vi "VisualizeStatus.vi"(10 "ModuleList":string[](array[string])=["Sync", "FGen", "Digitizer", "Sensor", "Analysis", "Scope", "AcPwr"]) -> ()   [LabVIEW 2018, in "Visualization.lvlib" / "VisualizeStatus.lvclass"]
uses:
  VisualizeStatus.lvclass
  VisualizeBase/VisualizeBase_class/SubVIs/VisualizationOptions.ctl
  <vilib>/Utility/miscctls.llb/LVRectTypeDef.ctl
  LV_Config_class/Config.lvclass/Config.ctl
  LV_Config_class/Typedefs/eLogLvl.ctl
  <vilib>/Utility/error.llb/DialogType.ctl
  VisualizeBase/VisualizeBase_class/Requests/VisUserEventType.ctl
  <vilib>/event_ctls.llb/usereventprio.ctl
  LV_Config_class/Accessors/Read ConfigFilePath.vi
  <extravilib>/ChannelInstances/Tag-bool/Write With Abort.vi
  <extravilib>/ChannelInstances/Tag-bool/Read With Abort.vi
  <vilib>/Utility/error.llb/Error Cluster From Error Code.vi
  <extravilib>/ChannelInstances/Tag-bool/Instantiate.vi
  <extravilib>/ChannelInstances/Tag-bool/EndpointRead.vi
  <userlib>/_OpenG.lib/string/string.llb/Convert EOLs (String)__ogtk.vi
  <extravilib>/ChannelInstances/Tag-bool/Endpoint.vi
  <vilib>/ErrorRing/Error Ring.xnode
  <userlib>/NIST/NISTErrorLib/NISTErrorLib.lvlib
  VisualizeBase/VisualizeBase_class/VisualizeBase.lvclass
  Sync/SyncModule/SyncModule.lvlib
  Digitizer/DigitizerModule/DigitizerModule.lvlib
  BusClass/Bus.lvclass
  Sensor/SensorModule/SensorModule.lvlib
  Analysis/AnalysisModule/AnalysisModule.lvlib
  Scope/ScopeModule/ScopeModule.lvlib
  AcPwr/AcPwrShared/AcPwrShared.lvlib
  <extravilib>/ChannelInstances/Tag-bool.lvlib
  TestClass/Test.lvclass
  FGen/FgenShared/FgenShared.lvlib
  LV_Config_class/Config.lvclass
panel:
  in  "Text.Scroll Position":i32=-1
  out "VisualizationProperties":T1={"PauseAtStartup"=TRUE, "LogData"=FALSE, "LaunchInSubPanel"=TRUE, "FPMonitor"=0, "FPWindowBounds"={"Left"=0, "Top"=0, "Right"=0, "Bottom"=0}, "MonitorBounds"={"Left"=0, "Top"=0, "Right"=0, "Bottom"=0}, "MeasIndices"=[]}
  out "Status Message":string
  in  "INIFilePath":path
  in  "Log Data":bool
  out "ErrorArray":errorcluster[](array[cluster])
  in  "btnRestart":bool
  in  "btnPause":bool
  in  "btnReset":bool
  in  "btnClear":bool
  in  "btnStop&Exit":bool
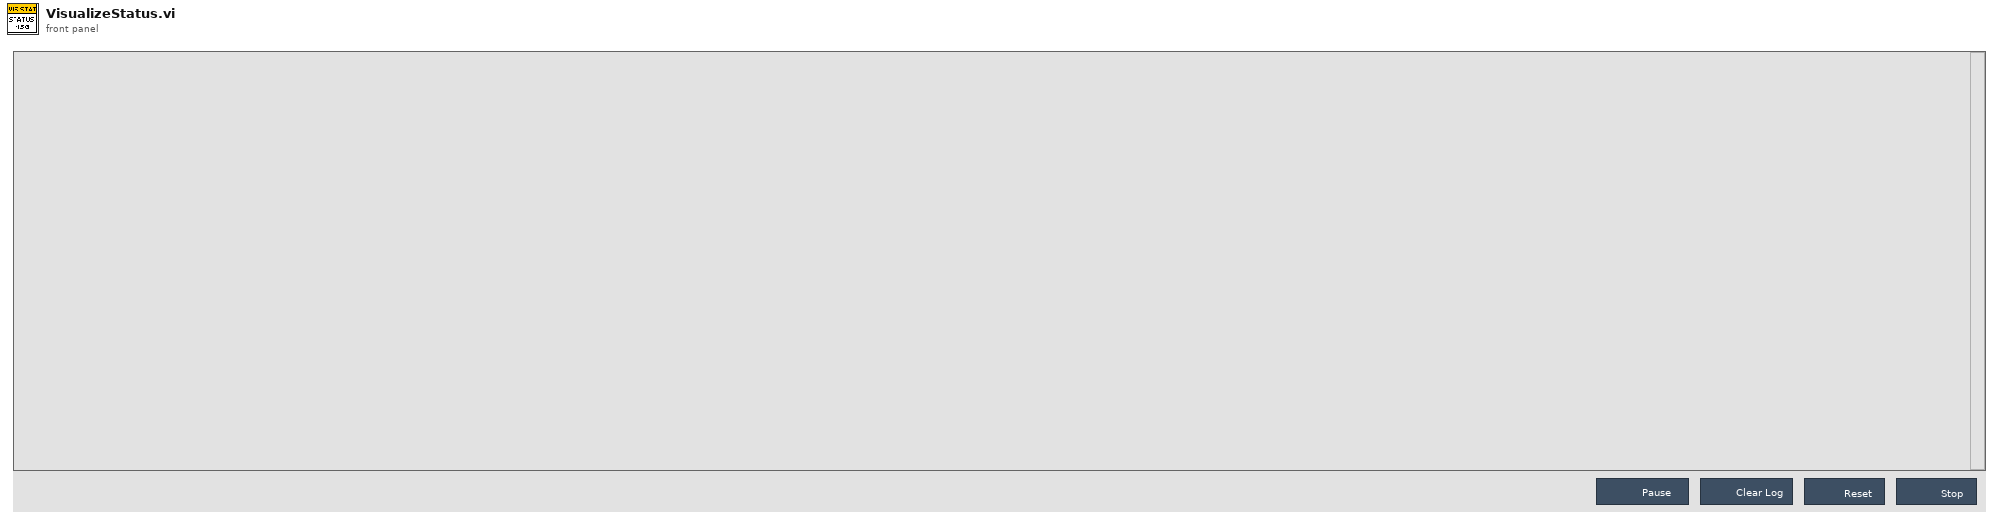
[diagram p1: front panel]
types:
  T1 = typedef "Visualization.lvlib/VisualizeBase.lvclass/VisualizationOptions.ctl" = cluster{"PauseAtStartup":bool, "LogData":bool, "LaunchInSubPanel":bool, "FPMonitor":u16, "FPWindowBounds":T2, "MonitorBounds":cluster{"Left":i16, "Top":i16, "Right":i16, "Bottom":i16}, "MeasIndices":i32[]}
  T2 = typedef "LVRectTypeDef.ctl" = cluster{"Left":i16, "Top":i16, "Right":i16, "Bottom":i16}
  T3 = typedef "SyncModule.lvlib/SyncBroadcastEvents.ctl" = cluster{"DidInit":refnum<user-event>, "StatusUpdate":refnum<user-event>, "ErrorReport":refnum<user-event>, "DidStop":refnum<user-event>, "PathToINI":refnum<user-event>, "TriggerTime":refnum<user-event>, "LockStatus":refnum<user-event>, "Info":refnum<user-event>, "ClockProperties":refnum<user-event>, "SyncData":refnum<user-event>, "TimingSession":refnum<user-event>}
  T4 = typedef "AcPwrShared.lvlib/AcPwrBroadcastEvents.ctl" = cluster{"DidInit":refnum<user-event>, "StatusUpdate":refnum<user-event>, "ErrorReport":refnum<user-event>, "DidStop":refnum<user-event>, "PathToINI":refnum<user-event>, "Measurements":refnum<user-event>, "LoadConfigFile":refnum<user-event>, "GetSettings":refnum<user-event>, "SetSettings":refnum<user-event>, "GetType&ID":refnum<user-event>, "GotSettings":refnum<user-event>, "GotSettingsLV":refnum<user-event>, "ParameterSet":refnum<user-event>}
  T5 = typedef "FgenShared.lvlib/clBroadcastEvents.ctl" = cluster{"DidInit":refnum<user-event>, "StatusUpdate":refnum<user-event>, "ErrorReport":refnum<user-event>, "DidStop":refnum<user-event>, "PathToINI":refnum<user-event>, "Channels":refnum<user-event>, "Function":refnum<user-event>, "Waveforms":refnum<user-event>, "Triggers":refnum<user-event>, "FunctionParams":refnum<user-event>, "FunctionArbs":refnum<user-event>, "FunctionSampleRate":refnum<user-event>}
  T6 = typedef "ScopeShared.lvlib/clBroadcastEvents.ctl" = cluster{"DidInit":refnum<user-event>, "StatusUpdate":refnum<user-event>, "ErrorReport":refnum<user-event>, "DidStop":refnum<user-event>, "PathToINI":refnum<user-event>, "Handle":refnum<user-event>, "Model":refnum<user-event>, "Channels":refnum<user-event>, "Acquisition":refnum<user-event>, "Trigger":refnum<user-event>, "ExtAcquisition":refnum<user-event>, "Waveform":refnum<user-event>}
  T7 = typedef "DigitizerShared.lvlib/clBroadcastEvents.ctl" = cluster{"DidInit":refnum<user-event>, "StatusUpdate":refnum<user-event>, "ErrorReport":refnum<user-event>, "DidStop":refnum<user-event>, "PathToINI":refnum<user-event>, "Channels":refnum<user-event>, "Acq":refnum<user-event>, "Trigger":refnum<user-event>, "Waveforms":refnum<user-event>}
  T8 = typedef "SensorShared.lvlib/clBroadcastEvents.ctl" = cluster{"DidInit":refnum<user-event>, "StatusUpdate":refnum<user-event>, "ErrorReport":refnum<user-event>, "DidStop":refnum<user-event>, "PathToINI":refnum<user-event>, "SensorReport":refnum<user-event>, "SensorConfig":refnum<user-event>}
  T9 = typedef "AnalysisModule.lvlib/clBroadcastEvents.ctl" = cluster{"DidInit":refnum<user-event>, "StatusUpdate":refnum<user-event>, "ErrorReport":refnum<user-event>, "DidStop":refnum<user-event>, "PathToINI":refnum<user-event>, "Config":refnum<user-event>, "ResultReport":refnum<user-event>, "FunctionClass":refnum<user-event>, "State":refnum<user-event>, "FunctionParams":refnum<user-event>, "Duration":refnum<user-event>}
  T10 = cluster{"DigitizerEvents":T7, "FGenEvents":T5, "SyncBroadcastEvents":T3, "AnalysisBroadcastEvents":T9, "SensorBdcstEvents":T8, "ScopeEvents":T6, "clAcPwrEvents":T4}
  T11 = typedef "Visualization.lvlib/VisualizeBase.lvclass/VisRequestEvents.ctl" = cluster{"StopRequest":refnum<user-event>, "ResetRequest":refnum<user-event>, "FP Pop In or Out":refnum<user-event>}
  T12 = cluster{"StatusUpdate":refnum<user-event>, "ErrorReport":refnum<user-event>, "StatusUpdate":refnum<user-event>, "ErrorReport":refnum<user-event>, "StatusUpdate":refnum<user-event>, "ErrorReport":refnum<user-event>, "StatusUpdate":refnum<user-event>, "ErrorReport":refnum<user-event>, "StatusUpdate":refnum<user-event>, "ErrorReport":refnum<user-event>, "StatusUpdate":refnum<user-event>, "ErrorReport":refnum<user-event>, "FunctionClass":refnum<user-event>, "StatusUpdate":refnum<user-event>, "ErrorReport":refnum<user-event>}
  T13 = typedef "Visualization.lvlib/VisualizeBase.lvclass/VisFrmWrkBroadcastEvents.ctl" = cluster{"StatusUpdate":refnum<user-event>, "DidStop":refnum<user-event>, "NewModuleLoaded":refnum<user-event>, "StopVisualization":refnum<user-event>}
  T14 = typedef "Visualization.lvlib/VisualizeBase.lvclass/VisUserEventType.ctl" = cluster{"BusIndex":i8, "Data":variant}
  T15 = typedef "usereventprio.ctl" = enum32{"high priority", "normal priority"}
  T16 = typedef "Tag-bool.lvlib/))Channel.ctl" = refnum<queue>
  T17 = typedef "Config_class.lvlib/Config.lvclass/eLogLvl.ctl" = enum16{"Normal", "Verbose", "None"}
  T18 = typedef "DialogType.ctl" = u16
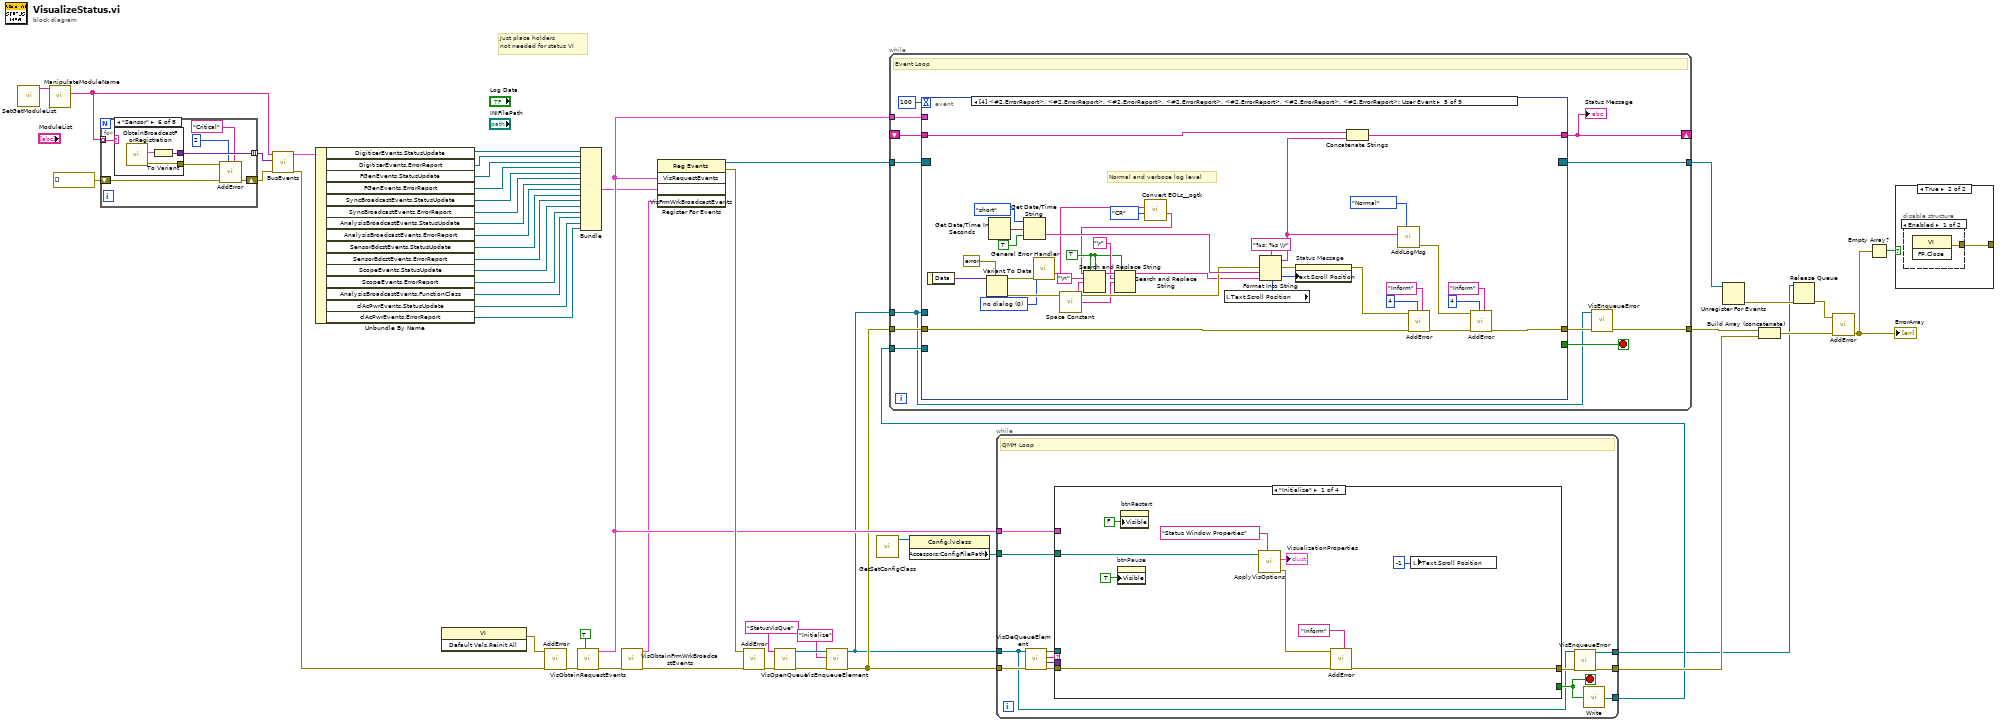
[diagram p0: block diagram]
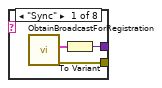
[diagram p2: hidden frame]
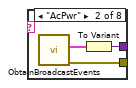
[diagram p3: hidden frame]
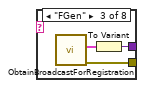
[diagram p4: hidden frame]
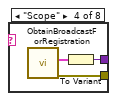
[diagram p5: hidden frame]
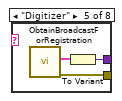
[diagram p6: hidden frame]
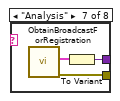
[diagram p7: hidden frame]
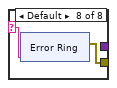
[diagram p8: hidden frame]
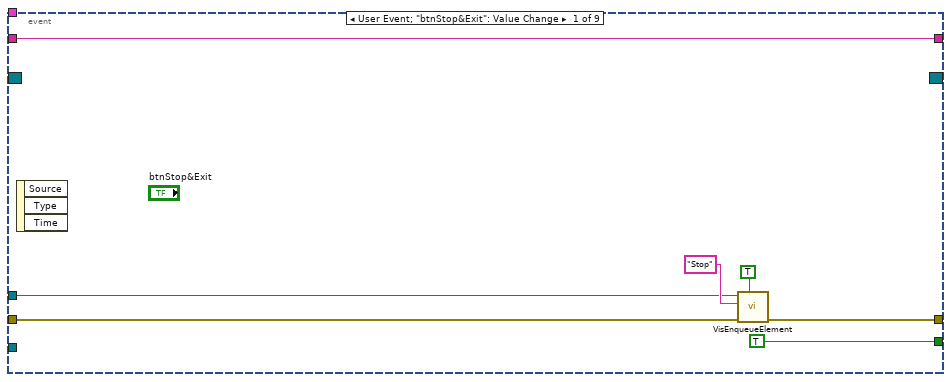
[diagram p9: hidden frame]
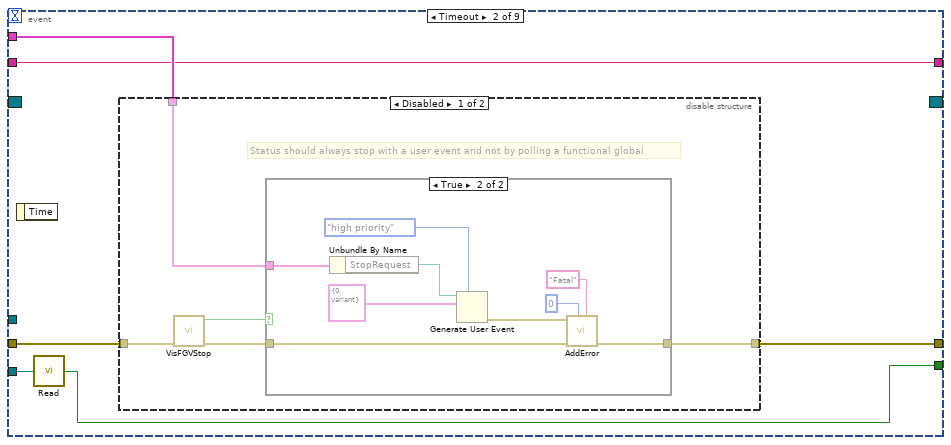
[diagram p10: hidden frame]
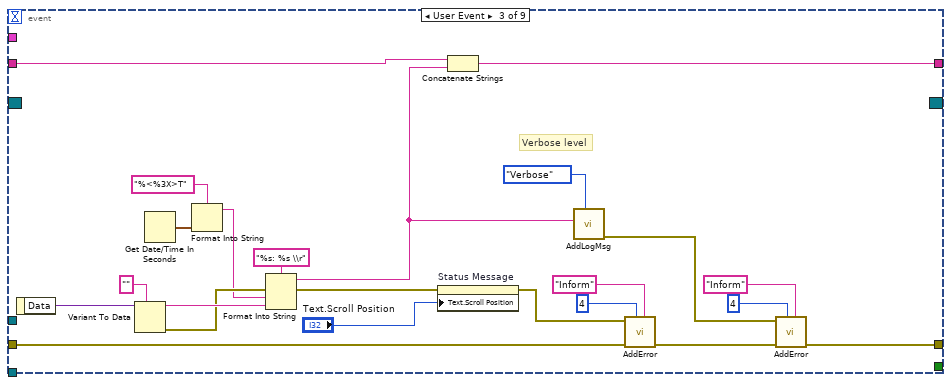
[diagram p13: hidden frame]
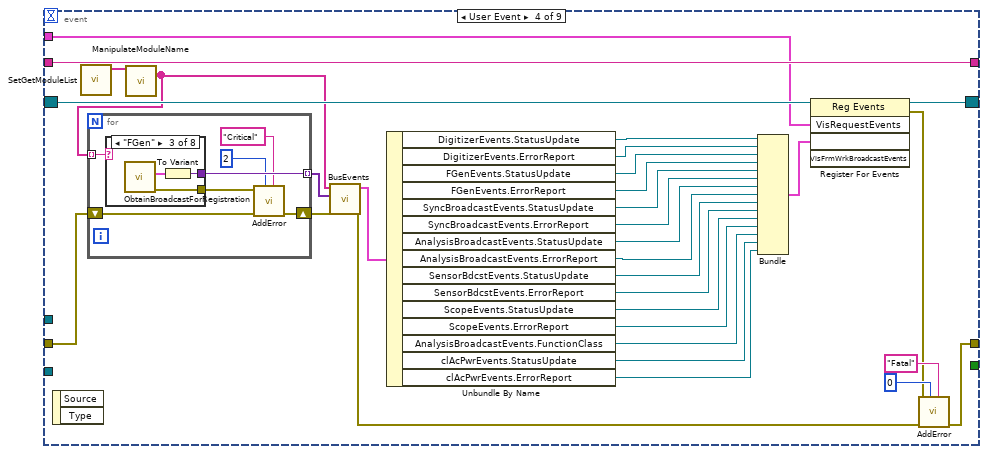
[diagram p14: hidden frame]
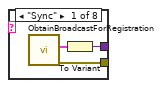
[diagram p15: hidden frame]
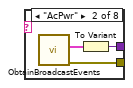
[diagram p16: hidden frame]
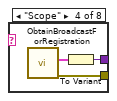
[diagram p17: hidden frame]
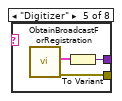
[diagram p18: hidden frame]
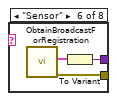
[diagram p19: hidden frame]
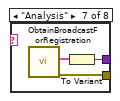
[diagram p20: hidden frame]
diagram:
  # "Just place holders\nnot needed for status VI"
  n1 = call "SetGetModuleList.vi"() -> ("ModuleList"=w35:string[])  [unwired: 11 in]
  n2 = call "ManipulateModuleName.vi"("ModuleListArrayIn"=w35) -> ("BeforeMatch:ModuleListArray"=w31:string[])  [unwired: 9 in, 5 out]
  n3 = for {
    shift-right: [w56] -> w33
    shift-left: errorcluster[] [] ("ErrorArray") -> [w55]
    tunnel: [w54] -> w32 mode=indexing
    tunnel: w31 -> [w51] mode=indexing
    n4 = case shown="\"Sensor\"" w51 {
      selector: w51 -> [_ _ _ _ _ _ _ w79]
      tunnel: [w59 w63 w65 w67 w71 w74 w77 _] -> w54
      tunnel: [w58 w62 w66 w69 w72 w75 w78 w80] -> w57
      frame "Sync" {
        n5 = call "ObtainBroadcastForRegistration.vi"() -> ("error out"=w58:errorcluster, "SyncBroadcastEvents"=w60:T3)  [unwired: 10 in]
        n6 = To Variant(anything=w60) -> (Variant=w59:variant)
      }
      frame "AcPwr" {
        n7 = call "ObtainBroadcastEvents.vi"() -> ("error out"=w62:errorcluster, "AcPwrEvents"=w61:T4)  [unwired: 10 in]
        n8 = To Variant(anything=w61) -> (Variant=w63:variant)
      }
      frame "FGen" {
        n9 = call "ObtainBroadcastForRegistration.vi"() -> ("error out"=w66:errorcluster, "FgenBroadcastEvents"=w64:T5)  [unwired: 10 in]
        n10 = To Variant(anything=w64) -> (Variant=w65:variant)
      }
      frame "Scope" {
        n11 = call "ObtainBroadcastForRegistration.vi"() -> ("error out"=w69:errorcluster, "ScopeBroadcastEvents"=w68:T6)  [unwired: 10 in]
        n12 = To Variant(anything=w68) -> (Variant=w67:variant)
      }
      frame "Digitizer" {
        n13 = call "ObtainBroadcastForRegistration.vi"() -> ("error out"=w72:errorcluster, "clDigitizerBdcstEvents"=w70:T7)  [unwired: 10 in]
        n14 = To Variant(anything=w70) -> (Variant=w71:variant)
      }
      frame "Sensor" {
        n15 = call "ObtainBroadcastForRegistration.vi"() -> ("error out"=w75:errorcluster, "SensorBdcstEvents"=w73:T8)  [unwired: 10 in]
        n16 = To Variant(anything=w73) -> (Variant=w74:variant)
      }
      frame "Analysis" {
        n17 = call "ObtainBroadcastForRegistration.vi"() -> ("error out"=w78:errorcluster, "AnalysisBroadcastEvents"=w76:T9)  [unwired: 10 in]
        n18 = To Variant(anything=w76) -> (Variant=w77:variant)
      }
      frame Default {
        n19 = xnode "Error Ring"("parameter 0"=w79) -> ("error out"=w80:errorcluster)
      }
    }
    n20 = call <userlib>:"AddError.vi"("Severity"="Critical", "Priority"=u8 2, "ErrorArray In"=w55, "error in (no error)"=w57) -> ("ErrorArray Out"=w56:errorcluster[])  [unwired: 6 in, 1 out]
  }
  n21 = call "BusEvents.vi"("Error in"=w33, "EventArray"=w32, "ModuleList"=w31) -> ("output cluster"=w30:T10)  [unwired: 7 in, 1 out]
  n22 = Unbundle By Name(w30) -> ("DigitizerEvents.StatusUpdate"=w29:refnum<user-event>, "DigitizerEvents.ErrorReport"=w28:refnum<user-event>, "FGenEvents.StatusUpdate"=w27:refnum<user-event>, "FGenEvents.ErrorReport"=w26:refnum<user-event>, "SyncBroadcastEvents.StatusUpdate"=w25:refnum<user-event>, "SyncBroadcastEvents.ErrorReport"=w24:refnum<user-event>, "AnalysisBroadcastEvents.StatusUpdate"=w23:refnum<user-event>, "AnalysisBroadcastEvents.ErrorReport"=w22:refnum<user-event>, "SensorBdcstEvents.StatusUpdate"=w21:refnum<user-event>, "SensorBdcstEvents.ErrorReport"=w20:refnum<user-event>, "ScopeEvents.StatusUpdate"=w19:refnum<user-event>, "ScopeEvents.ErrorReport"=w18:refnum<user-event>, "AnalysisBroadcastEvents.FunctionClass"=w17:refnum<user-event>, "clAcPwrEvents.StatusUpdate"=w16:refnum<user-event>, "clAcPwrEvents.ErrorReport"=w15:refnum<user-event>)
  n23 = invoke class="VI" method="Default Vals.Reinit All"() -> (error out=w50:errorcluster)  [unwired: 3 in, 2 out]
  n24 = call <userlib>:"AddError.vi"("ErrorArray In"=w33, "error in (no error)"=w50) -> ("ErrorArray Out"=w49:errorcluster[])  [unwired: 8 in, 1 out]
  n25 = call "VisObtainRequestEvents.vi"("Set (T)/Get (F)"=TRUE, "Error"=w49) -> ("Error"=w48:errorcluster[], "VisRequestEvents"=w36:T11)  [unwired: 8 in]
  n26 = Bundle("StatusUpdate"=w29, "ErrorReport"=w28, "StatusUpdate"=w27, "ErrorReport"=w26, "StatusUpdate"=w25, "ErrorReport"=w24, "StatusUpdate"=w23, "ErrorReport"=w22, "StatusUpdate"=w21, "ErrorReport"=w20, "StatusUpdate"=w19, "ErrorReport"=w18, "FunctionClass"=w17, "StatusUpdate"=w16, "ErrorReport"=w15) -> (w14:T12)  [unwired: 1 in]
  n27 = call "VisObtainFrmWrkBroadcastEvents.vi"("Error"=w48) -> ("Error"=w12:errorcluster[], "VisFrmWrkBroadcastEvents"=w11:T13)  [unwired: 9 in]
  n28 = register-events(w36, w14, w11) -> (reference out=w40:refnum<event-registration>, error out=w39:errorcluster)  [unwired: 2 in]
  n29 = call <userlib>:"AddError.vi"("ErrorArray In"=w12, "error in (no error)"=w39) -> ("ErrorArray Out"=w5:errorcluster[])  [unwired: 8 in, 1 out]
  n30 = call "VisOpenQueue.vi"("Error Array In"=w5, "QueueName"="StatusVisQue" ("QueName")) -> ("Error Array Out"=w7:errorcluster[], "queue out"=w8:refnum<queue>)  [unwired: 8 in]
  n31 = call "VisEnqueueElement.vi"("Error Array In"=w7, "Message"="Initialize", "queue in"=w8) -> ("Error Array Out"=w4:errorcluster[], "queue out"=w3:refnum<queue>)  [unwired: 7 in]
  n32 = call "GetSetConfigClass.vi"() -> ("Ref out"=w10:refnum<class "Config.lvclass">)  [unwired: 11 in]
  n33 = property class="Config.lvclass"(reference=w10) -> ("Accessors:ConfigFilePath"=w9:path)  [unwired: 1 in, 2 out]
  n34 = while {
    tunnel: w4 -> [w100]
    tunnel: [w94] -> w45
    tunnel: w36 -> [w93]
    tunnel: [w92] -> w37
    tunnel: w9 -> [w91]
    tunnel: w3 -> [w89]
    tunnel: [w88] -> w1
    stop <- w95 stop-if-true
    # "QMH Loop"
    n35 = call "VisDeQueueElement.vi"("Error Array In"=w100, "Queue In"=w89) -> ("Error Array Out"=w97:errorcluster[], "Data"=w98:variant, "Message"=w99:string, "Queue Out"=w90:refnum<queue>)  [unwired: 6 in]
    n36 = case shown="\"Initialize\"" w99 {
      selector: w99 -> [_ w117 _ _]
      tunnel: w98 -> [_ _ w132 _]
      tunnel: w97 -> [w110 w115 _ w164]
      tunnel: [w107 w114 w128 w162] -> w96
      tunnel: [_ _ w127 TRUE] -> w95
      tunnel: w93 -> [_ _ w126 _]
      tunnel: w91 -> [w109 _ _ w159]
      tunnel: w90 -> [_ _ w125 _]
      frame "Initialize" {
        n37 = property on="btnPause" class="Bool"("Visible"=TRUE) -> ()  [unwired: 2 in, 2 out]
        n38 = property on="btnRestart" class="Bool"("Visible"=FALSE) -> ()  [unwired: 2 in, 2 out]
        n39 = call "ApplyVisOptions.vi"("section (optional)"="Status Window Properties", "INIFilePath"=w109) -> ("error out"=w106:errorcluster, "VisualizationProperties"=→"VisualizationProperties":T1)  [unwired: 8 in]
        n40 = call <userlib>:"AddError.vi"("Severity"="Inform", "ErrorArray In"=w110, "error in (no error)"=w106) -> ("ErrorArray Out"=w107:errorcluster[])  [unwired: 7 in, 1 out]
        n41 = local write "Text.Scroll Position"(-1 ("Text.Scroll Position")) -> ()
      }
      frame Default {
        n42 = xnode "Error Ring"("parameter 0"=w117) -> ("error out"=w116:errorcluster)
        n43 = call <userlib>:"AddError.vi"("Severity"="Inform" ("String"), "Priority"=u8 5, "ErrorArray In"=w115, "error in (no error)"=w116) -> ("ErrorArray Out"=w114:errorcluster[], "error out"=w113:errorcluster)  [unwired: 6 in]
        n44 = call <vilib>:"Clear Errors.vi"("error in (no error)"=w113) -> ()  [unwired: 5 in, 2 out]
      }
      frame "Error" {
        n45 = Variant To Data(type=errorcluster[] [], Variant=w132) -> (data=w130:errorcluster[])  [unwired: 1 in, 1 out]
        n46 = call <userlib>:"ParseErrors.vi"("ErrorArray"=w130) -> ("ErrorArray"=w129:errorcluster[])  [unwired: 8 in, 2 out]
        n47 = for {
          tunnel: w129 -> [w143] mode=indexing
          tunnel: [w137] -> w128 mode=concatenating
          tunnel: [w135] -> w127
          tunnel: w126 -> [w134]
          tunnel: w125 -> [w133]
          stop <- w135 stop-if-true
          n48 = call <userlib>:"GeneralHandler.vi"("error in (no error)"=w143) -> ("Severity"=w136:string, "Stop"=w140:bool, "Abort"=w141:bool, "Continue"=w142:bool)  [unwired: 6 in, 1 out]
          n49 = Build Array(w142, w141, w140) -> (w139:bool[])
          n50 = Boolean Array To Number(Boolean array=w139) -> (number=w138:u32)
          n51 = case shown="2" w138 {
            tunnel: [_ _ w148 w156] -> w137
            tunnel: w136 -> [_ _ _ w152]
            tunnel: [_ _ _ w150] -> w135
            tunnel: w134 -> [_ _ _ w149]
            tunnel: w133 -> [_ _ w144 _]
            frame 0, Default {
              # "No Dialog"
            }
            frame 1 {
              # "Continue"
            }
            frame 2 {
              # "Abort, Flush Queue"
              n52 = Flush Queue(queue=w144) -> (error out=w147:errorcluster)  [unwired: 1 in, 2 out]
              n53 = call <userlib>:"AddError.vi"("Severity"="Critical" ("String"), "Priority"=u8 1, "error in (no error)"=w147) -> ("ErrorArray Out"=w148:errorcluster[])  [unwired: 7 in, 1 out]
            }
            frame 4 {
              # "Stop"
              n54 = Unbundle By Name(w149) -> ("StopRequest"=w157:refnum<user-event>)
              n55 = Equal?(x="Fatal", y=w152) -> (x = y?=w150:bool)
              n56 = Generate User Event(priority (normal)=usereventprio."high priority", user event=w157, event data cluster=T14 {"BusIndex"=0, "Data"=variant} ("event data")) -> (error out=w155:errorcluster)  [unwired: 1 in, 1 out]
              n57 = call <userlib>:"AddError.vi"("error in (no error)"=w155) -> ("ErrorArray Out"=w156:errorcluster[])  [unwired: 9 in, 1 out]
            }
          }
        }
      }
      frame "Stop" {
        n58 = local read "VisualizationProperties"() -> (w158:T1)
        n59 = call "WriteVisOptionsToINIFile.vi"("section (optional)"="Status Window Properties", "Visualization Options"=w158, "INIFilePath"=w159) -> ("error out"=w161:errorcluster)  [unwired: 7 in, 1 out]
        n60 = call <userlib>:"AddError.vi"("Severity"="Inform", "ErrorArray In"=w164, "error in (no error)"=w161) -> ("ErrorArray Out"=w162:errorcluster[])  [unwired: 7 in, 1 out]
      }
    }
    n61 = call "VisEnqueueError.vi"("Error Array In"=w96, "Queue in"=w89) -> ("Error Array Out"=w94:errorcluster[], "Queue out"=w88:refnum<queue>)  [unwired: 8 in]
    n62 = call <extravilib>:"Write.vi"("element"=w95) -> ("channel"=w92:T16)  [unwired: 1 out]
  }
  n63 = while {
    tunnel: w40 -> [w177]
    tunnel: [w174] -> w46
    tunnel: [w173] -> w47
    tunnel: w36 -> [w172]
    shift-right: [w169] -> _
    shift-left: _ -> [w171]
    tunnel: w4 -> [w170]
    tunnel: w37 -> [w167]
    tunnel: w3 -> [w166]
    stop <- w176 stop-if-true
    # "Event Loop"
    n64 = event shown="[4] <#2.ErrorReport>, <#2.ErrorReport>, <#2.ErrorReport>, <#2.ErrorReport>, <#2.ErrorReport>, <#2.ErrorReport>, <#2.ErrorReport>: User Event" {
      selector: w177 -> [_ _ _ w255 _ _ _ _ _]
      dyn-events: [_ _ _ w257 _ _ _ _ _] -> w173
      timeout: 100 -> [_ _ _ _ _ _ _ _ _]
      tunnel: [TRUE w185 _ _ _ _ _ _ _] -> w176
      tunnel: [w183 w190 w211 w260 w311 _ w336 _ _] -> w175
      tunnel: w172 -> [_ w188 _ w248 _ _ w335 _ _]
      tunnel: [w179 w187 w223 w253 w320 "" w333 w343 w348] -> w169
      tunnel: w171 -> [w179 w187 w222 w253 w319 _ w333 w343 w348]
      tunnel: w170 -> [w180 w189 w221 w254 w317 _ w334 _ _]
      tunnel: w167 -> [_ w186 _ _ _ _ _ _ _]
      tunnel: w166 -> [w178 _ _ _ _ _ _ _ _]
      event User Event; "btnStop&Exit": Value Change {
        n65 = event-data() -> ()  [unwired: 1 in, 3 out]
        n66 = call "VisEnqueueElement.vi"("Priority? (F)"=TRUE, "Error Array In"=w180, "Message"="Stop", "queue in"=w178) -> ("Error Array Out"=w183:errorcluster[])  [unwired: 6 in, 1 out]
      }
      event Timeout {
        n67 = event-data() -> ()  [unwired: 1 in, 1 out]
        n68 = call <extravilib>:"Read.vi"("channel"=w186) -> ("element"=w185:bool)  [unwired: 1 in, 1 out]
        n69 = disable-structure shown="Disabled" {
          disable-tunnel: [w194 w206] -> w190
          disable-tunnel: w189 -> [w193 w206]
          disable-tunnel: w188 -> [w191 _]
          frame Disabled {
            # "Status should always stop with a user event and not by polling a functional global"
            n70 = call "VisFGVStop.vi"("Error In"=w193) -> ("Error Out"=w192:errorcluster[], "Value"=w195:bool)  [unwired: 9 in]
            n71 = case shown="True" w195 {
              tunnel: [w196 w199] -> w194
              tunnel: w192 -> [w196 w198]
              tunnel: w191 -> [_ w197]
              frame False {
              }
              frame True {
                n72 = Unbundle By Name(w197) -> ("StopRequest"=w205:refnum<user-event>)
                n73 = Generate User Event(priority (normal)=usereventprio."high priority", user event=w205, event data cluster=T14 {"BusIndex"=0, "Data"=variant} ("event data")) -> (error out=w200:errorcluster)  [unwired: 1 in, 1 out]
                n74 = call <userlib>:"AddError.vi"("Severity"="Fatal" ("String"), "Priority"=u8 0, "ErrorArray In"=w198, "error in (no error)"=w200) -> ("ErrorArray Out"=w199:errorcluster[])  [unwired: 6 in, 1 out]
              }
            }
          }
          frame Enabled {
          }
        }
      }
      event User Event {
        # "Verbose level"
        n75 = event-data() -> ("Data"=w217:variant)  [unwired: 1 in]
        n76 = Variant To Data(type="", Variant=w217) -> (data=w227:string, error out=w226:errorcluster)  [unwired: 1 in]
        n77 = Get Date/Time In Seconds() -> (seconds since 1Jan1904=w209:timestamp)
        n78 = Format Into String(format string="%<%3X>T", w209) -> (resulting string=w208:string)  [unwired: 2 in, 1 out]
        n79 = Format Into String(format string="%s: %s \\r", error in=w226, w208, w227) -> (resulting string=w216:string, error out=w220:errorcluster)  [unwired: 1 in]
        n80 = property on="Status Message" class="Str"(error in=w220, "Text.Scroll Position"="Text.Scroll Position") -> (error out=w219:errorcluster)  [unwired: 1 in, 1 out]
        n81 = Concatenate Strings(w222, w216) -> (w223:string)
        n82 = call "AddLogMsg.vi"("LogLevel"=eLogLvl."Verbose", "LogMsg"=w216) -> ("error out"=w213:errorcluster)  [unwired: 9 in]
        n83 = call <userlib>:"AddError.vi"("Severity"="Inform", "Priority"=u8 4, "ErrorArray In"=w221, "error in (no error)"=w219) -> ("ErrorArray Out"=w212:errorcluster[])  [unwired: 6 in, 1 out]
        n84 = call <userlib>:"AddError.vi"("Severity"="Inform", "Priority"=u8 4, "ErrorArray In"=w212, "error in (no error)"=w213) -> ("ErrorArray Out"=w211:errorcluster[])  [unwired: 6 in, 1 out]
      }
      event User Event {
        n85 = event-data() -> ()  [unwired: 1 in, 2 out]
        n86 = call "SetGetModuleList.vi"() -> ("ModuleList"=w252:string[])  [unwired: 11 in]
        n87 = call "ManipulateModuleName.vi"("ModuleListArrayIn"=w252) -> ("BeforeMatch:ModuleListArray"=w230:string[])  [unwired: 9 in, 5 out]
        n88 = for {
          shift-right: [w266] -> w249
          shift-left: w254 -> [w265]
          tunnel: [w264] -> w251 mode=indexing
          tunnel: w230 -> [w261] mode=indexing
          n89 = case shown="\"FGen\"" w261 {
            selector: w261 -> [_ _ _ _ _ _ _ w289]
            tunnel: [w269 w273 w275 w279 w281 w284 w287 _] -> w264
            tunnel: [w268 w272 w276 w278 w282 w285 w288 w290] -> w267
            frame "Sync" {
              n90 = call "ObtainBroadcastForRegistration.vi"() -> ("error out"=w268:errorcluster, "SyncBroadcastEvents"=w270:T3)  [unwired: 10 in]
              n91 = To Variant(anything=w270) -> (Variant=w269:variant)
            }
            frame "AcPwr" {
              n92 = call "ObtainBroadcastEvents.vi"() -> ("error out"=w272:errorcluster, "AcPwrEvents"=w271:T4)  [unwired: 10 in]
              n93 = To Variant(anything=w271) -> (Variant=w273:variant)
            }
            frame "FGen" {
              n94 = call "ObtainBroadcastForRegistration.vi"() -> ("error out"=w276:errorcluster, "FgenBroadcastEvents"=w274:T5)  [unwired: 10 in]
              n95 = To Variant(anything=w274) -> (Variant=w275:variant)
            }
            frame "Scope" {
              n96 = call "ObtainBroadcastForRegistration.vi"() -> ("error out"=w278:errorcluster, "ScopeBroadcastEvents"=w277:T6)  [unwired: 10 in]
              n97 = To Variant(anything=w277) -> (Variant=w279:variant)
            }
            frame "Digitizer" {
              n98 = call "ObtainBroadcastForRegistration.vi"() -> ("error out"=w282:errorcluster, "clDigitizerBdcstEvents"=w280:T7)  [unwired: 10 in]
              n99 = To Variant(anything=w280) -> (Variant=w281:variant)
            }
            frame "Sensor" {
              n100 = call "ObtainBroadcastForRegistration.vi"() -> ("error out"=w285:errorcluster, "SensorBdcstEvents"=w283:T8)  [unwired: 10 in]
              n101 = To Variant(anything=w283) -> (Variant=w284:variant)
            }
            frame "Analysis" {
              n102 = call "ObtainBroadcastForRegistration.vi"() -> ("error out"=w288:errorcluster, "AnalysisBroadcastEvents"=w286:T9)  [unwired: 10 in]
              n103 = To Variant(anything=w286) -> (Variant=w287:variant)
            }
            frame Default {
              n104 = xnode "Error Ring"("parameter 0"=w289) -> ("error out"=w290:errorcluster)
            }
          }
          n105 = call <userlib>:"AddError.vi"("Severity"="Critical", "Priority"=u8 2, "ErrorArray In"=w265, "error in (no error)"=w267) -> ("ErrorArray Out"=w266:errorcluster[])  [unwired: 6 in, 1 out]
        }
        n106 = call "BusEvents.vi"("Error in"=w249, "EventArray"=w251, "ModuleList"=w230) -> ("Error out"=w250:errorcluster[], "output cluster"=w247:T10)  [unwired: 7 in]
        n107 = Unbundle By Name(w247) -> ("DigitizerEvents.StatusUpdate"=w246:refnum<user-event>, "DigitizerEvents.ErrorReport"=w245:refnum<user-event>, "FGenEvents.StatusUpdate"=w244:refnum<user-event>, "FGenEvents.ErrorReport"=w243:refnum<user-event>, "SyncBroadcastEvents.StatusUpdate"=w242:refnum<user-event>, "SyncBroadcastEvents.ErrorReport"=w241:refnum<user-event>, "AnalysisBroadcastEvents.StatusUpdate"=w240:refnum<user-event>, "AnalysisBroadcastEvents.ErrorReport"=w239:refnum<user-event>, "SensorBdcstEvents.StatusUpdate"=w238:refnum<user-event>, "SensorBdcstEvents.ErrorReport"=w237:refnum<user-event>, "ScopeEvents.StatusUpdate"=w236:refnum<user-event>, "ScopeEvents.ErrorReport"=w235:refnum<user-event>, "AnalysisBroadcastEvents.FunctionClass"=w234:refnum<user-event>, "clAcPwrEvents.StatusUpdate"=w233:refnum<user-event>, "clAcPwrEvents.ErrorReport"=w232:refnum<user-event>)
        n108 = Bundle("StatusUpdate"=w246, "ErrorReport"=w245, "StatusUpdate"=w244, "ErrorReport"=w243, "StatusUpdate"=w242, "ErrorReport"=w241, "StatusUpdate"=w240, "ErrorReport"=w239, "StatusUpdate"=w238, "ErrorReport"=w237, "StatusUpdate"=w236, "ErrorReport"=w235, "FunctionClass"=w234, "StatusUpdate"=w233, "ErrorReport"=w232) -> (w231:T12)  [unwired: 1 in]
        n109 = register-events(reference=w255, w248, w231) -> (reference out=w257:refnum<event-registration>, error out=w256:errorcluster)  [unwired: 2 in]
        n110 = call <userlib>:"AddError.vi"("Severity"="Fatal", "Priority"=u8 0, "ErrorArray In"=w250, "error in (no error)"=w256) -> ("ErrorArray Out"=w260:errorcluster[])  [unwired: 6 in, 1 out]
      }
      event User Event {
        w302 = TRUE ("replace all? (F)")
        w307 = T18 0 items=["no dialog", "OK message", "continue or stop message", "OK message + warnings", "continue/stop + warnings"] ("type of dialog (OK msg:1)")
        # "Normal and verbose log level"
        n111 = event-data() -> ("Data"=w328:variant)  [unwired: 1 in]
        n112 = Variant To Data(type=errorcluster {"status"=FALSE, "code"=0, "source"=""} ("error constant"), Variant=w328) -> (data=w308:errorcluster, error out=w325:errorcluster)  [unwired: 1 in]
        n113 = Get Date/Time In Seconds() -> (seconds since 1Jan1904=w331:timestamp)
        n114 = Get Date/Time String(date format (0)=enum16{"short", "long", "abbreviated"}."short", seconds (now)=w331, want seconds? (F)=TRUE) -> (time string=w326:string)  [unwired: 1 out]
        n115 = call <vilib>:"General Error Handler.vi"("type of dialog (OK msg:1)"=w307, "error in (no error)"=w308) -> ("message"=w298:string)  [unwired: 9 in, 4 out]
        n116 = call <vilib>:"Space Constant.vi"() -> ("String"=w303:string)
        n117 = call-poly <userlib>:"Convert EOLs__ogtk.vi"("Convert to:"=enum16{"CR", "LF", "CRLF"}."CR", "String in"=w298) -> ("String out"=w300:string)  [unwired: 9 in]
        n118 = Search and Replace String(replace all?=w302, case sensitive?=w302, input string=w300, search string="\n", replace string=w303) -> (result string=w305:string)  [unwired: 3 in, 3 out]
        n119 = Search and Replace String(replace all?=w302, input string=w305, search string="\r", replace string=w303) -> (result string=w299:string)  [unwired: 4 in, 3 out]
        n120 = local read "Text.Scroll Position"() -> (w309:i32)
        n121 = Format Into String(format string="%s: %s \\r", error in=w325, w326, w299) -> (resulting string=w310:string, error out=w324:errorcluster)  [unwired: 1 in]
        n122 = property on="Status Message" class="Str"(error in=w324, "Text.Scroll Position"=w309) -> (error out=w323:errorcluster)  [unwired: 1 in, 1 out]
        n123 = Concatenate Strings(w319, w310) -> (w320:string)
        n124 = call "AddLogMsg.vi"("LogLevel"=eLogLvl."Normal", "LogMsg"=w310) -> ("error out"=w313:errorcluster)  [unwired: 9 in]
        n125 = call <userlib>:"AddError.vi"("Severity"="Inform", "Priority"=u8 4, "ErrorArray In"=w317, "error in (no error)"=w323) -> ("ErrorArray Out"=w312:errorcluster[])  [unwired: 6 in, 1 out]
        n126 = call <userlib>:"AddError.vi"("Severity"="Inform", "Priority"=u8 4, "ErrorArray In"=w312, "error in (no error)"=w313) -> ("ErrorArray Out"=w311:errorcluster[])  [unwired: 6 in, 1 out]
      }
      event "btnClear": Value Change {
        n127 = event-data() -> ()  [unwired: 1 in, 1 out]
      }
      event "btnReset": Value Change {
        n128 = event-data() -> ()  [unwired: 1 in, 1 out]
        n129 = Unbundle By Name(w335) -> ("ResetRequest"=w337:refnum<user-event>)
        n130 = Generate User Event(priority (normal)=usereventprio."high priority", user event=w337, event data cluster=T14 {"BusIndex"=0, "Data"=variant} ("event data")) -> (error out=w340:errorcluster)  [unwired: 1 in, 1 out]
        n131 = call <userlib>:"AddError.vi"("Severity"="Fatal", "Priority"=u8 0, "ErrorArray In"=w334, "error in (no error)"=w340) -> ("ErrorArray Out"=w336:errorcluster[])  [unwired: 6 in, 1 out]
      }
      event "btnPause": Value Change {
        n132 = event-data() -> ()  [unwired: 1 in, 2 out]
        n133 = property on="Status Message" class="Str"() -> ("Text.Scroll Position"=w344:u32)  [unwired: 2 in, 2 out]
        n134 = property on="btnRestart" class="Bool"("Visible"=TRUE) -> ()  [unwired: 2 in, 2 out]
        n135 = local write "Text.Scroll Position"(w344) -> ()
        n136 = property on="btnPause" class="Bool"("Visible"=FALSE) -> ()  [unwired: 2 in, 2 out]
      }
      event "btnRestart": Value Change {
        w347 = -1 ("Text.Scroll Position")
        n137 = event-data() -> ()  [unwired: 1 in, 2 out]
        n138 = property on="btnRestart" class="Bool"("Visible"=FALSE) -> ()  [unwired: 2 in, 2 out]
        n139 = local write "Text.Scroll Position"(w347) -> ()
        n140 = property on="btnPause" class="Bool"("Visible"=TRUE) -> ()  [unwired: 2 in, 2 out]
        n141 = property on="Status Message" class="Str"("Text.Scroll Position"=w347) -> ()  [unwired: 2 in, 2 out]
      }
    }
    "Status Message" <- w169
    n142 = call "VisEnqueueError.vi"("Error Array In"=w175, "Queue in"=w166) -> ("Error Array Out"=w174:errorcluster[])  [unwired: 8 in, 1 out]
  }
  n143 = Unregister For Events(event registration refnum=w47) -> (error out=w44:errorcluster)  [unwired: 1 in]
  n144 = Build Array (concatenate)(w46, w45) -> (w43:errorcluster[])
  n145 = Release Queue(queue=w1, error in (no error)=w44) -> (error out=w42:errorcluster)  [unwired: 1 in, 2 out]
  n146 = call <userlib>:"AddError.vi"("ErrorArray In"=w43, "error in (no error)"=w42) -> ("ErrorArray Out"=w13:errorcluster[])  [unwired: 8 in, 1 out]
  "ErrorArray" <- w13
  n147 = Empty Array?(array=w13) -> (empty?=w41:bool)
  n148 = case shown="True" w41 {
    tunnel: [_ w351] -> _
    frame False {
    }
    frame True {
      n149 = disable-structure shown="Enabled" {
        disable-tunnel: [w352 _] -> w351
        frame Enabled {
          n150 = invoke class="VI" method="FP.Close"() -> (error out=w352:errorcluster)  [unwired: 3 in, 2 out]
        }
        frame Disabled {
        }
      }
    }
  }
